vi "Intensity Graphs to Excel.vi"(9 "RIGHT":dbl[][](graph)=array100x100[10000 elements], 11 "LEFT":dbl[][](graph)=array100x100[10000 elements]) -> ()   [LabVIEW 2013]
panel:
  out "Right":string
  out "Left":string
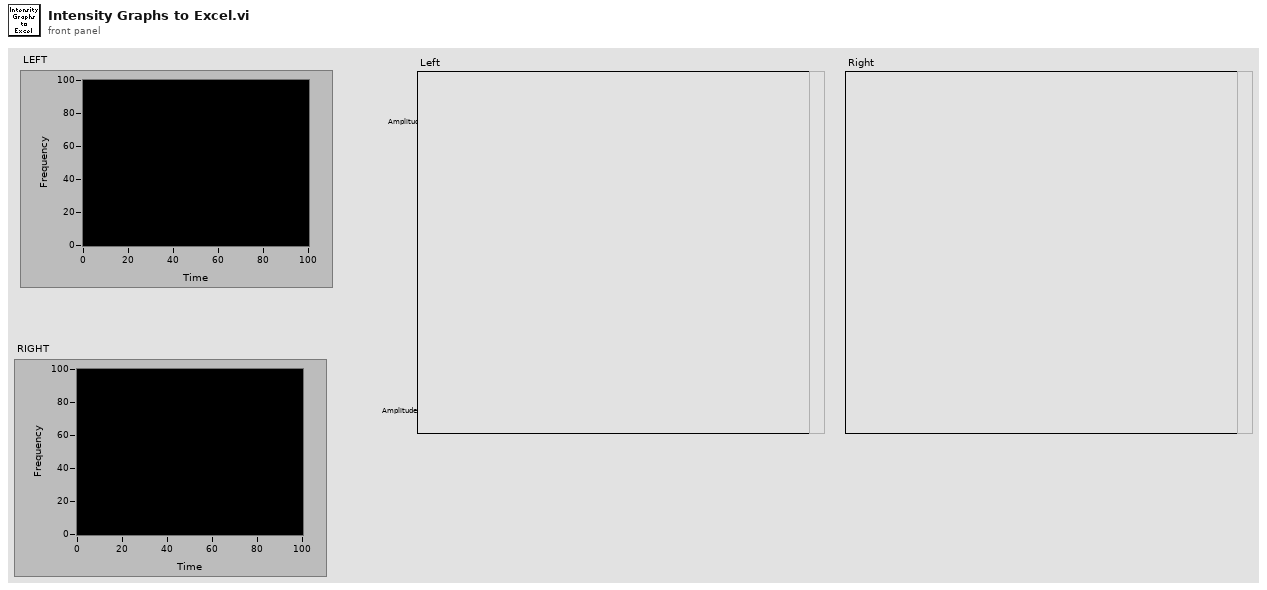
[diagram p1: front panel]
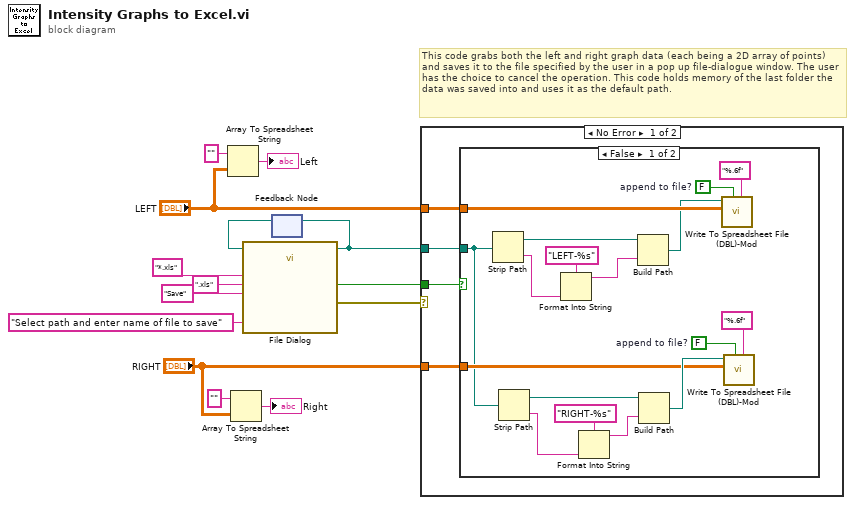
[diagram p0: block diagram]
diagram:
  # "This code grabs both the left and right graph data (each being a 2D array of points) and saves it to the file specified by the user in a pop up file-dialogue window. The user has the choice to cancel the operation. This code holds memory of the last folder the data was saved into and uses it as the default path."
  n1 = Array To Spreadsheet String(array="LEFT", 3:"" ("format string")) -> (spreadsheet string=→"Left":string)  [unwired: 1 in]
  n2 = Array To Spreadsheet String(array="RIGHT", 3:"" ("format string")) -> (spreadsheet string=→"Right":string)  [unwired: 1 in]
  n3 = feedback #1() -> (w9:path)  [unwired: 1 in]
  n4 = call "File Dialog"("start path"=w9, "prompt"="Select path and enter name of file to save", "button label"="Save", "pattern (all files)"="*.xls" ("pattern label"), "pattern label"=".xls") -> ("selected path"=w4:path, "cancelled"=w10:bool, "error out"=w11:errorcluster)  [unwired: 7 in, 1 out]
  n5 = feedback-in #1(w4) -> ()
  n6 = case shown="No Error" w11 {
    tunnel: "LEFT" -> [w18 _]
    tunnel: w10 -> [w17 _]
    tunnel: w4 -> [w16 _]
    tunnel: "RIGHT" -> [w15 _]
    frame No Error {
      n7 = case shown="False" w17 {
        tunnel: w18 -> [w35 _]
        tunnel: w16 -> [w21 _]
        tunnel: w15 -> [w22 _]
        frame False {
          w19 = FALSE  # append to file?
          w20 = FALSE  # append to file?
          n8 = Strip Path(path=w21) -> (stripped path=w31:path, name=w32:string)
          n9 = Strip Path(path=w21) -> (stripped path=w26:path, name=w25:string)
          n10 = Format Into String(format string="LEFT-%s", w32) -> (resulting string=w30:string)  [unwired: 2 in, 1 out]
          n11 = Format Into String(format string="RIGHT-%s", w25) -> (resulting string=w27:string)  [unwired: 2 in, 1 out]
          n12 = Build Path(base path=w31, name or relative path=w30) -> (appended path=w29:path)
          n13 = Build Path(base path=w26, name or relative path=w27) -> (appended path=w28:path)
          n14 = call "Write To Spreadsheet File (DBL)-Mod.vi"("format (%.3f)"="%.6f", "append to file? (new file:F)"=w19, "2D data"=w35, "file path (dialog if empty)"=w29) -> ()  [unwired: 6 in, 2 out]
          n15 = call "Write To Spreadsheet File (DBL)-Mod.vi"("format (%.3f)"="%.6f", "append to file? (new file:F)"=w20, "2D data"=w22, "file path (dialog if empty)"=w28) -> ()  [unwired: 6 in, 2 out]
        }
        frame True {
        }
      }
    }
    frame Error {
    }
  }
